vi "Icon_Remove Border from 2D image.vi"(8 "Error":errorcluster, 11 "2D Image":T1) -> (0 "Error Out":errorcluster, 3 "Border Removed Out":T1)   [LabVIEW 2009]
uses:
  Controls/Array/Color Box Array_2D Icon Viewer.ctl
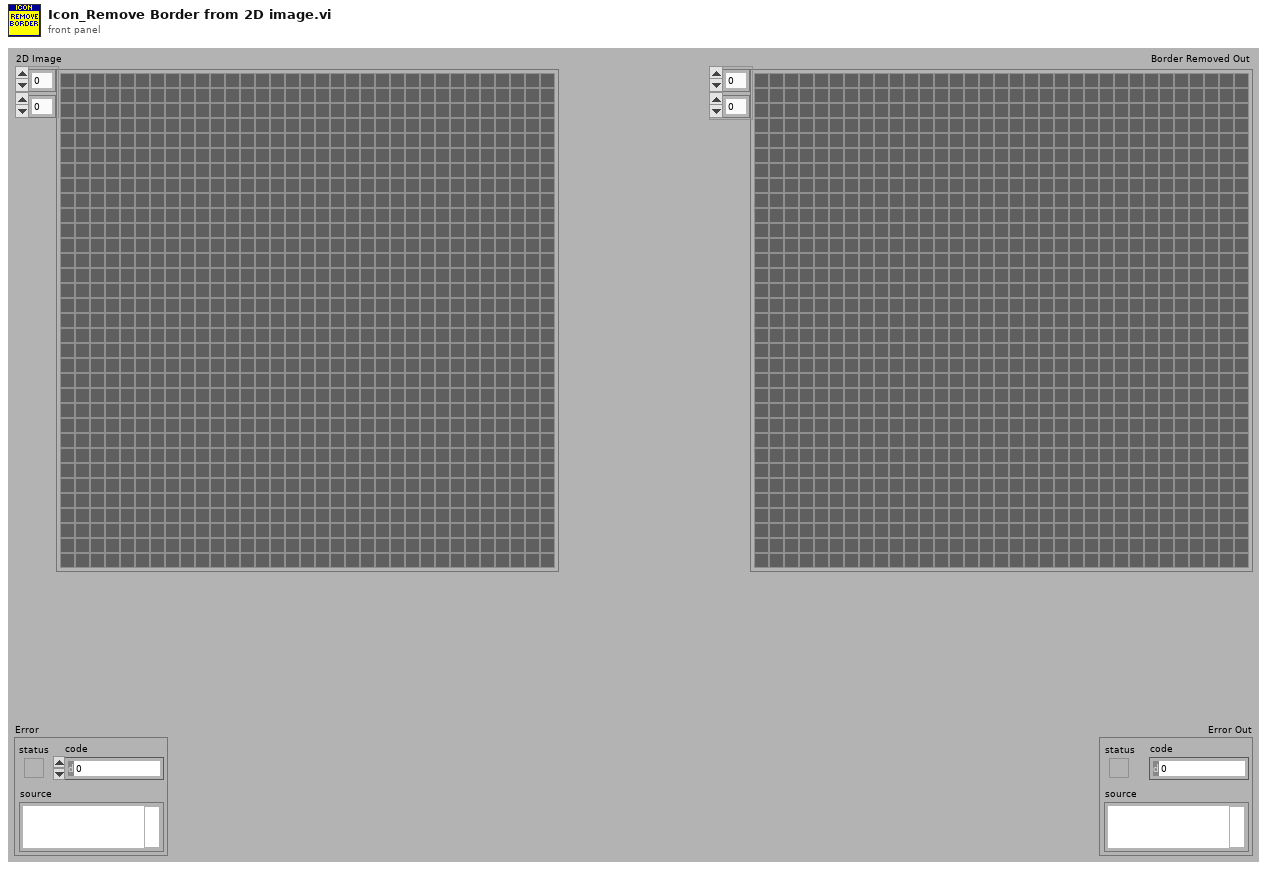
[diagram p1: front panel]
types:
  T1 = typedef "Color Box Array_2D Icon Viewer.ctl" = u32[][]
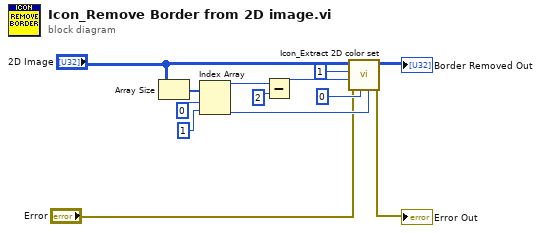
[diagram p0: block diagram]
diagram:
  n1 = Array Size(array="2D Image") -> (size(s)=w8:i32[])
  n2 = Index Array(array=w8, index #1=0 ("index"), index #2=1 ("index")) -> (element #1=w6:i32, element #2=w2:i32)
  n3 = Subtract(x=w6, y=2) -> (x-y=w3:i32)
  n4 = call "Icon_Extract 2D color set.vi"("Width"=w2, "Left"=0, "Error"="Error", "Height"=w3, "Top"=1, "2D Image"="2D Image") -> ("Error Out"=→"Error Out":errorcluster, "2D Image Out"=→"Border Removed Out":T1)  [unwired: 4 in]
